vi "SetComment.vi"(8 "error in":errorcluster, 10 "Comment":string, 11 "UserComment in":refnum<class "UserComment.lvclass">) -> (0 "error out":errorcluster, 3 "UserComment out":refnum<class "UserComment.lvclass">)   [LabVIEW 2021, in "ProligentXMLGenerator.lvlib" / "UserComment.lvclass"]
doc: "This value will be truncated by the DIT if longer than 255 characters.\nNote that whitespaces at the end of any strings will be discarded."
uses:
  UserComment.lvclass
  UserComment.lvclass/UserComment.ctl
  Base/NonNullableString_TruncateAt_255/NonNullableString_TruncateAt_255.lvclass
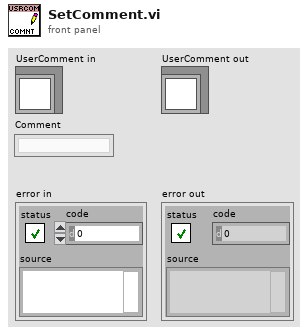
[diagram p1: front panel]
types:
  T1 = typedef "ProligentXMLGenerator.lvlib/UserComment.lvclass/Data.ctl" = cluster{"Name":string, "Comment":refnum<class "NonNullableString_TruncateAt_255.lvclass">, "User":refnum<class "NonEmptyString_255.lvclass">, "Time":refnum<class "DateTime.lvclass">}
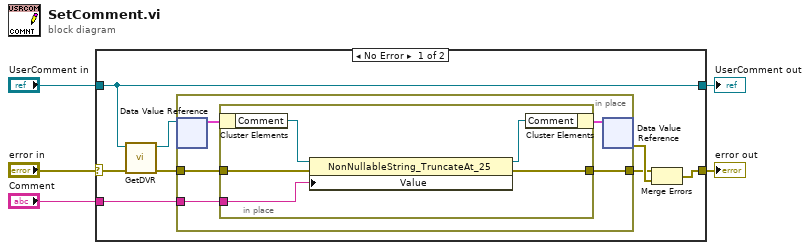
[diagram p0: block diagram]
diagram:
  n1 = case shown="No Error" "error in" {
    selector: "error in" -> [w11 w24]
    tunnel: "UserComment in" -> [w6 w25]
    tunnel: [w8 w24] -> w3
    tunnel: "Comment" -> [w7 _]
    tunnel: [w6 w25] -> w1
    frame No Error {
      n2 = call "GetDVR.vi"("error in"=w11, "UserComment"=w6) -> ("error out"=w10:errorcluster, "DVRReference"=w12:refnum<data-value>)  [unwired: 8 in]
      n3 = in-place "In Place Element Structure" {
        in-place-border: w10 -> [w18]
        in-place-border: [w17] -> w9
        in-place-border: w7 -> [w16]
        n4 = in-place-dvr #1(w12) -> (w15:T1)  [unwired: 1 out]
        n5 = in-place {
          in-place-border: w18 -> [w23]
          in-place-border: [w22] -> w17
          in-place-border: w16 -> [w21]
          n6 = in-place-cluster #2(w15) -> ("Comment"=w20:refnum<class "NonNullableString_TruncateAt_255.lvclass">)
          n7 = property on="Property Node" class="NonNullableString_TruncateAt_25"(reference=w20, error in=w23, "Value"=w21) -> (reference out=w19:refnum<class "NonNullableString_TruncateAt_255.lvclass">, error out=w22:errorcluster)
          n8 = in-place-cluster #2("Comment"=w19) -> (w14:T1)
        }
        n9 = in-place-dvr #1(w14) -> (w13:errorcluster)  [unwired: 1 out]
      }
      n10 = Merge Errors(w9, w13) -> (w8:errorcluster)
    }
    frame Error {
    }
  }
  "error out" <- w3
  "UserComment out" <- w1
